vi "array to waveform.vi"(6 "reset events":T1(array[cluster]), 9 "dataset ID":u16, 10 "num samples in dataset":u32, 11 "array dataset":i32[][](array[numeric])) -> (2 "cleared array dataset out":i32[][](array[numeric]), 3 "waveform dataset":waveform(dbl)[](array[waveform]))   [LabVIEW 2017]
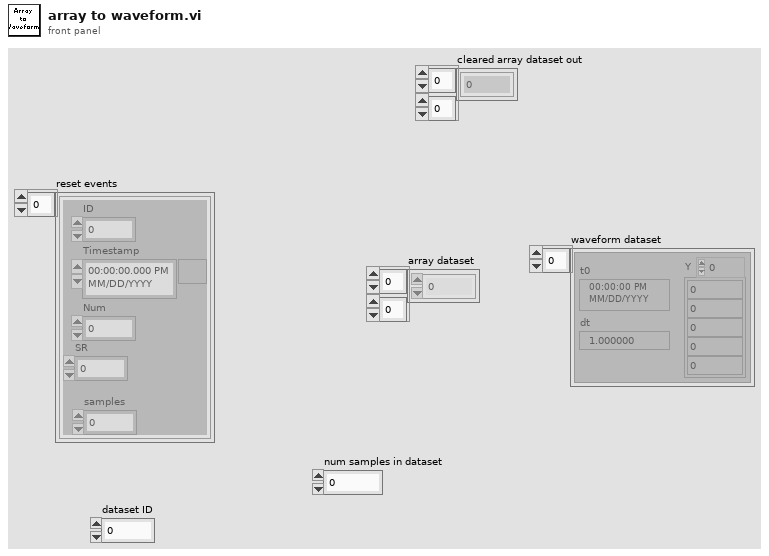
[diagram p1: front panel]
types:
  T1 = cluster{"ID":u16, "Timestamp":timestamp, "Num":u16, "SR":dbl, "samples":u16}[]
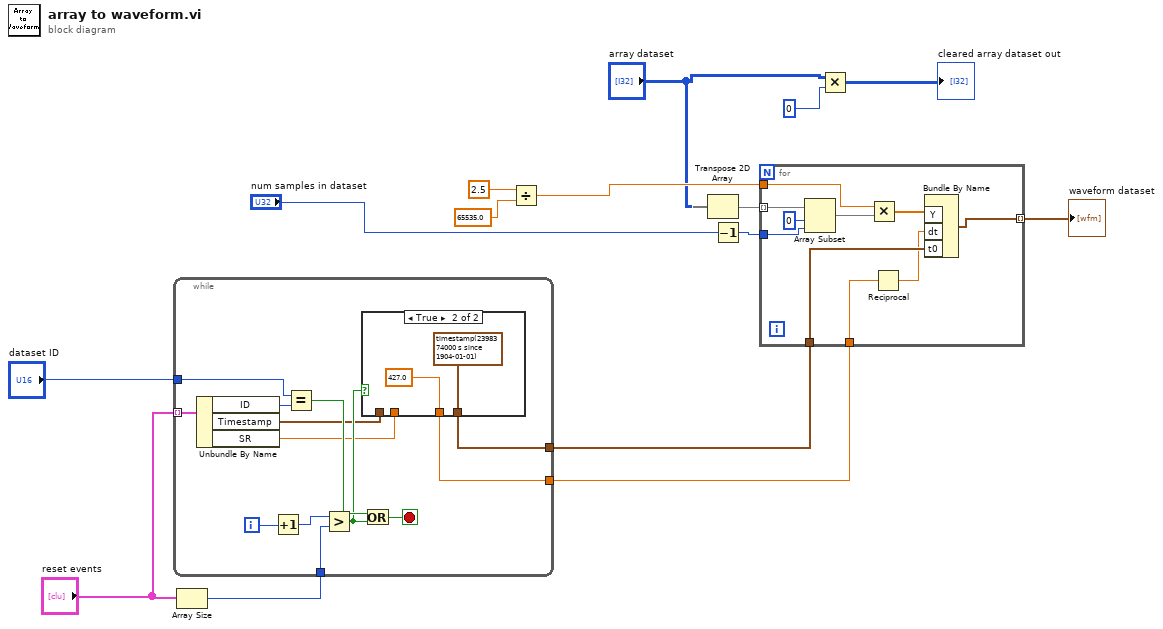
[diagram p0: block diagram]
diagram:
  n1 = Array Size(array="reset events") -> (size(s)=w12:i32)
  n2 = while {
    tunnel: "reset events" -> [w28] mode=indexing
    tunnel: "dataset ID" -> [w26]
    tunnel: [w19] -> w13
    tunnel: w12 -> [w24]
    tunnel: [w16] -> w1
    i -> [w25]
    stop <- w22 stop-if-true
    n3 = Unbundle By Name(w28) -> ("ID"=w27:u16, "Timestamp"=w20:timestamp, "SR"=w17:dbl)
    n4 = Increment(x=w25) -> (x+1=w18:i32)
    n5 = Equal?(x=w26, y=w27) -> (x = y?=w23:bool)
    n6 = Greater?(x=w18, y=w24) -> (0:w21:bool)
    n7 = case shown="True" w21 {
      tunnel: w20 -> [w30 _]
      tunnel: [w30 timestamp(2398374000 s since 1904-01-01) ("Timestamp")] -> w19
      tunnel: [w29 427.0 ("SR")] -> w16
      tunnel: w17 -> [w29 _]
      frame False {
      }
      frame True {
      }
    }
    n8 = Or(x=w23, y=w21) -> (x .or. y?=w22:bool)
  }
  n9 = Divide(x=2.5 ("dt"), y=65535.0 ("dt")) -> (x/y=w9:dbl)
  n10 = Transpose 2D Array(2D array="array dataset") -> (transposed array=w15:i32[][])
  n11 = Decrement(x="num samples in dataset") -> (x-1=w14:u32)
  n12 = for {
    tunnel: w15 -> [w42] mode=indexing
    tunnel: w14 -> [w41]
    tunnel: w13 -> [w39]
    tunnel: [w36] -> w8 mode=indexing
    tunnel: w9 -> [w33]
    tunnel: w1 -> [w35]
    n13 = Array Subset(array=w42, index=0, length=w41) -> (w38:i32[])
    n14 = Multiply(x=w33, y=w38) -> (x*y=w37:dbl[])
    n15 = Reciprocal(x=w35) -> (1/x=w34:dbl)
    n16 = Bundle By Name("Y"=w37, "dt"=w34, "t0"=w39) -> (w36:waveform(dbl))  [unwired: 1 in]
  }
  "waveform dataset" <- w8
  n17 = Multiply(x="array dataset", y=0) -> (x*y=→"cleared array dataset out":i32[][])
